vi "Do.vi"(8 "error in (no error)":errorcluster, 10 "Actor In":refnum<class "Actor.lvclass">, 11 "Msg":refnum<class "Message Template.lvclass">) -> (0 "error out":errorcluster, 1 "Stop Actor":bool, 2 "Actor Out":refnum<class "Actor.lvclass">)   [LabVIEW 2020, in "Message Template.lvclass"]
uses:
  Message Template.lvclass
  Artifex/Actor/Actor.lvclass
  Artifex Template/Template/Template.lvclass
  C:/dev/lv20CE/relink/lv-artifex/Artifex/Actor/Actor.lvclass
  Message Template.lvclass/Message Template.ctl
  5e062f91-6507-428e-a57e-74783385ada6.vi
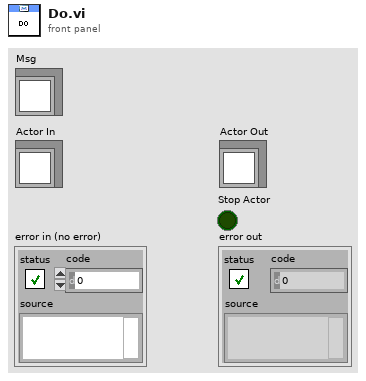
[diagram p1: front panel]
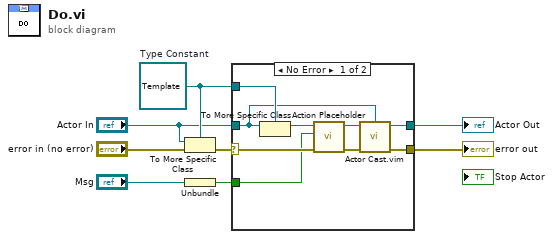
[diagram p0: block diagram]
diagram:
  w2 = refnum<class "Template.lvclass"> refnum  # Type Constant
  n1 = To More Specific Class(target class=w2, reference="Actor In", error in="error in (no error)") -> (error out=w3:errorcluster)  [unwired: 1 out]
  n2 = Unbundle("Msg") -> (w5:bool)
  n3 = case shown="No Error" w3 {
    selector: w3 -> [w17 w18]
    tunnel: [w13 w19] -> w8
    tunnel: [w10 w18] -> w7
    tunnel: w5 -> [w15 _]
    tunnel: w2 -> [w11 _]
    tunnel: "Actor In" -> [w9 w19]
    frame No Error {
      n4 = To More Specific Class(target class=w11, reference=w9) -> (specific class reference=w14:refnum<class "Template.lvclass">)  [unwired: 1 in, 1 out]
      n5 = call "Action Placeholder.vi"("error in (no error)"=w17, "Placeholder"=w15, "Actor In"=w14) -> ("error out"=w12:errorcluster, "Actor Out"=w16:refnum<class "Template.lvclass">)  [unwired: 7 in]
      n6 = call "Actor Cast.vim"("Type"=w9, "Actor in"=w16, "error in (no error)"=w12) -> ("Actor out"=w13:refnum<class "Actor.lvclass">, "error out"=w10:errorcluster)  [unwired: 6 in]
    }
    frame Error {
    }
  }
  "error out" <- w7
  "Actor Out" <- w8
